vi "Coerce I32 value.vi"(1 "upper limit (1000000000)":i32=1000000000, 2 "I32 value in":i32) -> (7 "Coerced value":i32)   [LabVIEW 2020]
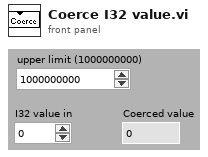
[diagram p1: front panel]
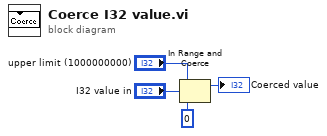
[diagram p0: block diagram]
diagram:
  n1 = In Range and Coerce(upper limit="upper limit (1000000000)", x="I32 value in", lower limit=0) -> (coerced(x)=→"Coerced value":i32)  [unwired: 1 out]
